vi "Read configuration.vi"(8 "error in (no error)":errorcluster, 11 "Abstract Engine in":refnum<class "Abstract Engine.lvclass">) -> (0 "error out":errorcluster, 2 "CEF_configuration":refnum<class "CEF_serializable configuration.lvclass">, 3 "Abstract Engine out":refnum<class "Abstract Engine.lvclass">)   [LabVIEW 2025, in "Abstract Engine.lvlib" / "Abstract Engine.lvclass"]
uses:
  Abstract Engine.lvclass
  Users/Public/Documents/Sandia National Labs/TSS Plugin/CEF.lvlibp/serializable configuration/CEF_serializable configuration.lvclass
  Abstract Engine.lvclass/Abstract Engine.ctl
  Engine configuration/Engine configuration.lvclass
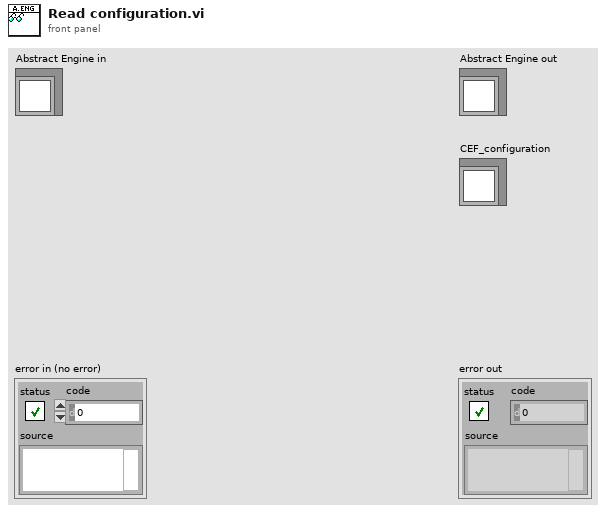
[diagram p1: front panel]
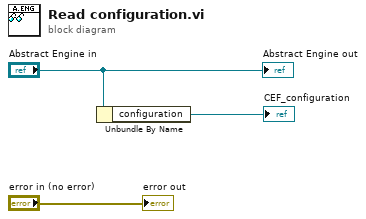
[diagram p0: block diagram]
diagram:
  n1 = Unbundle By Name("Abstract Engine in") -> ("configuration"=→"CEF_configuration":refnum<class "Engine configuration.lvclass">)
  "error out" <- "error in (no error)"
  "Abstract Engine out" <- "Abstract Engine in"
